vi "GetAssetChildren.vi"(8 "error in (no error)":errorcluster, 10 "parent id":string, 11 "service":refnum<class "IcmMessageService.lvclass">) -> (0 "error out":errorcluster, 3 "AssetNodes":T1[](array[typedef]))   [LabVIEW 2016]
doc: "Queries for all children of an asset node."
uses:
  <vilib>/addons/InsightCM/MessageBus/MessageService/IcmMessageService.lvclass
  <vilib>/addons/InsightCM/MessageBus/Base/controls/AssetNodeQueryParams.ctl
  <vilib>/addons/InsightCM/MessageBus/MessageLibrary/AssetManager/controls/AssetMgrQueryAssetNodeViewsRequestBody.ctl
  <vilib>/addons/InsightCM/MessageBus/Base/controls/AssetState.ctl
  <vilib>/addons/InsightCM/MessageBus/Base/controls/KeyValuePair.ctl
  <vilib>/addons/InsightCM/MessageBus/Base/controls/Metric.ctl
  <vilib>/addons/InsightCM/MessageBus/Base/controls/AssetNodeReference.ctl
  <vilib>/addons/InsightCM/MessageBus/Base/controls/AssetNodeView.ctl
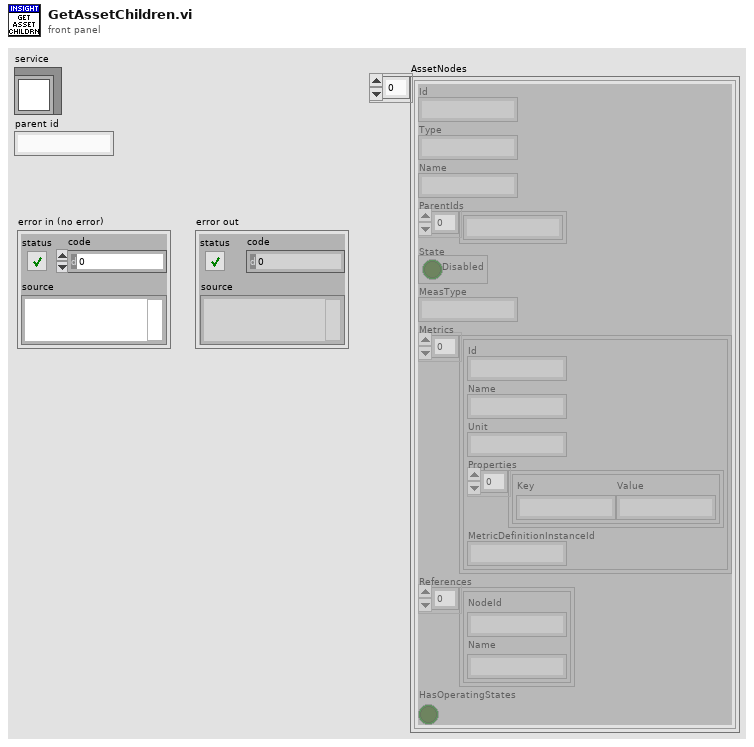
[diagram p1: front panel]
types:
  T1 = typedef "AssetNodeView.ctl" = cluster{"Id":string, "Type":string, "Name":string, "ParentIds":string[], "State":T2, "MeasType":string, "Metrics":T3[], "References":T5[], "HasOperatingStates":bool}
  T2 = typedef "AssetState.ctl" = cluster{"Disabled":bool}
  T3 = typedef "Metric.ctl" = cluster{"Id":string, "Name":string, "Unit":string, "Properties":T4[], "MetricDefinitionInstanceId":string}
  T4 = typedef "KeyValuePair.ctl" = cluster{"Key":string, "Value":string}
  T5 = typedef "AssetNodeReference.ctl" = cluster{"NodeId":string, "Name":string}
  T6 = typedef "AssetMgrQueryAssetNodeViewsRequestBody.ctl" = cluster{"QueryParams":T7}
  T7 = typedef "AssetNodeQueryParams.ctl" = cluster{"ViewType":string, "RootId":string, "IncludeRoot":bool, "Depth":i32, "SelectedNodes":string[]}
  T8 = typedef "Message.ctl" = cluster{"Header":T9, "Body":u8[]}
  T9 = typedef "MessageHeader.ctl" = cluster{"MessageName":string, "Timestamp":i64, "CorrelationId":string, "ContentType":string, "RoutingKey":string, "Properties":T4[]}
  T10 = typedef "AssetMgrQueryAssetNodeViewsResponseBody.ctl" = cluster{"AssetNodes":T1[]}
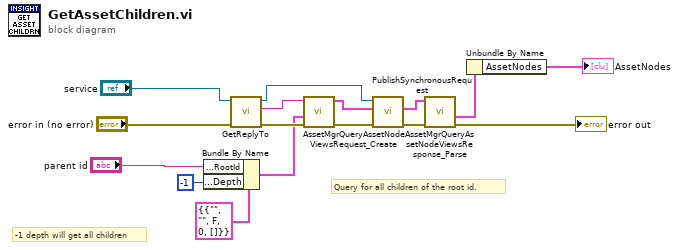
[diagram p0: block diagram]
diagram:
  # "-1 depth will get all children"
  # "Query for all children of the root id."
  n1 = Bundle By Name(cluster=T6 {"QueryParams"={"ViewType"="", "RootId"="", "IncludeRoot"=FALSE, "Depth"=0, "SelectedNodes"=[]}} ("AssetMgrQueryAssetNodeViewsRequest"), "QueryParams.RootId"="parent id", "QueryParams.Depth"=-1) -> (w2:T6)
  n2 = call <vilib>:"GetReplyTo.vi"("error in (no error)"="error in (no error)", "service in"="service") -> ("error out"=w6:errorcluster, "reply to"=w4:string, "service out"=w16:refnum<class "IcmMessageService.lvclass">)  [unwired: 7 in]
  n3 = call <vilib>:"AssetMgrQueryAssetNodeViewsRequest_Create.vi"("error in (no error)"=w6, "AssetMgrQueryAssetNodeViewsRequest"=w2, "ReplyTo"=w4) -> ("error out"=w5:errorcluster, "Message"=w1:T8)  [unwired: 7 in]
  n4 = call <vilib>:"PublishSynchronousRequest.vi"("error in (no error)"=w5, "request"=w1, "service in"=w16) -> ("error out"=w10:errorcluster, "response"=w7:T8)  [unwired: 6 in, 1 out]
  n5 = call <vilib>:"AssetMgrQueryAssetNodeViewsResponse_Parse.vi"("error in (no error)"=w10, "Message"=w7) -> ("error out"=→"error out":errorcluster, "Body"=w8:T10)  [unwired: 6 in, 2 out]
  n6 = Unbundle By Name(w8) -> ("AssetNodes"=→"AssetNodes":T1[])
